vi "inclination_from_gravity_vector.vi"(1 "Normalized gravity vector":dbl[](array[numeric])) -> (0 "Inclination (XZ, YZ)":dbl[](array[numeric]))   [LabVIEW 2015]
doc: "Calculates the angle in XZ (roll) and YZ (pitch) plane from the normalized gravity vector. The result is expressed in radians."
panel:
  out "angleYZ":dbl
  out "angleXZ":dbl
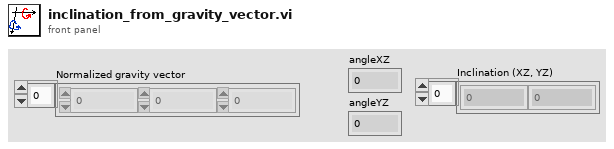
[diagram p1: front panel]
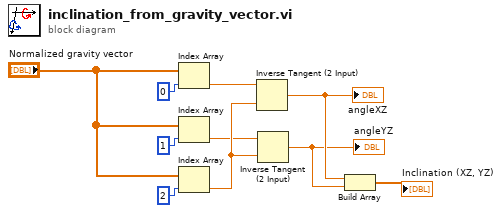
[diagram p0: block diagram]
diagram:
  n1 = Index Array "Index Array"(array="Normalized gravity vector", index=0) -> (element=w2:dbl)
  n2 = Index Array(array="Normalized gravity vector", index=1) -> (element=w1:dbl)
  n3 = Index Array(array="Normalized gravity vector", index=2) -> (element=w6:dbl)
  n4 = Inverse Tangent (2 Input)(1:w6, 2:w2) -> (0:w5:dbl)
  "angleXZ" <- w5
  n5 = Inverse Tangent (2 Input)(1:w6, 2:w1) -> (0:w4:dbl)
  "angleYZ" <- w4
  n6 = Build Array(w5, w4) -> (→"Inclination (XZ, YZ)":dbl[])
